vi "MLTraining.vi"(3 "model file (JSON)":path, 8 "Save model file as":string="model.json", 9 "model to train":T7(ring), 10 "Label setting":T2={"with label column?"=TRUE, "label column index"=-1}, 11 "training data file (CSV)":path) -> (0 "error out":errorcluster, 1 "feature trend":dbl[][](graph))   [LabVIEW 2017, in "MachineLearning.lvlib"]
doc: "Demonstrates how to find the optimal set of hyperparameters of the specific algorithm among SVM, Neural Network and Logistic Regression by grid search."
uses:
  MachineLearning.lvlib
  TypeDefs/Label Setting.ctl
  <vilib>/addons/AML/Classification/SVM/Controls/aml_SVM Grid Configuration.ctl
  <vilib>/addons/AML/Classification/SVM/Controls/aml_SVM Type.ctl
  <vilib>/addons/AML/Classification/SVM/Controls/aml_SVM Kernel Type.ctl
  <vilib>/addons/AML/Classification/Neural Network/Controls/aml_Neural Network Parameter Grid.ctl
  <vilib>/addons/AML/Classification/Neural Network/Controls/aml_Hidden Layer Type.ctl
  <vilib>/addons/AML/Classification/Neural Network/Controls/aml_Output Layer Type.ctl
  <vilib>/addons/AML/Classification/Neural Network/Controls/aml_NN Cost Function Type.ctl
  <vilib>/addons/AML/Classification/Logistic Regression/Controls/aml_Logistic Regression Parameters Grid.ctl
  <vilib>/addons/AML/Classification/SVM/Classes/AML SVM.lvclass/AML SVM.ctl
  <vilib>/addons/AML/Classification/Neural Network/Classes/AML Neural Network.lvclass/AML Neural Network.ctl
  <vilib>/addons/AML/Classification/Logistic Regression/Classes/AML Logistic Regression.lvclass/AML Logistic Regression.ctl
  <vilib>/addons/AML/Classification/SVM/Classes/aml_Read SVM Parameter.vi
  <vilib>/addons/AML/Classification/Neural Network/Classes/aml_Read Neural Network Parameter.vi
  <vilib>/addons/AML/Classification/Logistic Regression/Classes/aml_Read LR Parameters.vi
  <vilib>/addons/AML/Classification/SVM/Classes/AML SVM.lvclass
  C:/Program Files (x86)/National Instruments/LabVIEW 2017/vi.lib/addons/AML/Classification/Common/Classes/AML Classification.lvclass
  <vilib>/addons/AML/Classification/Neural Network/Classes/AML Neural Network.lvclass
  <vilib>/addons/AML/Classification/Logistic Regression/Classes/AML Logistic Regression.lvclass
  <vilib>/addons/AML/Classification/Initialize Classification Model (LR, Search).vi
  <vilib>/addons/AML/Classification/Initialize Classification Model (NN, Search).vi
  <vilib>/addons/AML/Classification/Initialize Classification Model (SVM, Search).vi
  <vilib>/addons/AML/Data/Load Training Data (2D Array).vi
  <vilib>/addons/AML/Analytics and Machine Learning.lvlib
panel:
  in  "Tab Control":T1(tab)
  in  "Tab Control 2":T3(tab)
  out "coef0":dbl
  out "gamma":dbl
  out "degree":i32
  out "nu":dbl
  out "c":dbl
  out "kernel type":enum32{"Linear", "Polynomial", "RBF", "Sigmoid"}(ring)
  out "SVM type":enum32{"C_SVC", "NU_SVC"}(ring)
  in  "hyperparameter optimization (SVM)":T4={"hyperparameter search method"=enum."Exhaustive search", "number of searchings"=1, "evaluation metric"=enum."Accuracy"} caption="hyperparameter optimization"
  in  "degree":i32[](array[numeric])=[3, 5]
  in  "nu":dbl[](array[numeric])=[0.3, 0.5]
  in  "c":dbl[](array[numeric])=[0.1, 1.0]
  in  "kernel type":T5(array[ring])=[enum."Linear", enum."Polynomial", enum."RBF", enum."Sigmoid"]
  in  "SVM type":enum32{"C_SVC", "NU_SVC"}[](array[ring])=[enum."C_SVC", enum."NU_SVC"]
  in  "gamma":dbl[](array[numeric])=[0.2, 0.5]
  in  "coef0":dbl[](array[numeric])=[0.0, 1.0]
  out "metrics (cross validation)":T6
  out "output layer type":enum16{"Sigmoid", "Softmax"}(ring)
  out "cost function type":enum16{"Quadratic", "Cross-entropy"}(ring)
  out "hidden layer type":enum16{"Sigmoid", "Tanh", "ReLU"}(ring)
  out "number of hidden neurons":i32
  in  "hyperparameter optimization (NN)":T4={"hyperparameter search method"=enum."Exhaustive search", "number of searchings"=1, "evaluation metric"=enum."Accuracy"} caption="hyperparameter optimization"
  in  "number of hidden neurons":i32[](array[numeric])=[5, 10]
  in  "hidden layer type":enum16{"Sigmoid", "Tanh", "ReLU"}[](array[ring])=[enum."Sigmoid", enum."Tanh", enum."ReLU"]
  in  "output layer type":enum16{"Sigmoid", "Softmax"}[](array[ring])=[enum."Sigmoid", enum."Softmax"]
  in  "cost function type":enum16{"Quadratic", "Cross-entropy"}[](array[ring])=[enum."Quadratic", enum."Cross-entropy"]
  out "metrics (cross validation)":T6
  out "max iteration":i32
  out "tolerance":dbl
  in  "tolerance":dbl[](array[numeric])=[0.001, 0.0001]
  in  "max iteration":i32[](array[numeric])=[500, 1000]
  in  "hyperparameter optimization (LR)":T4={"hyperparameter search method"=enum."Exhaustive search", "number of searchings"=1, "evaluation metric"=enum."Accuracy"} caption="hyperparameter optimization"
  out "metrics (cross validation)":T6
  # "Optimized Hyperparameters"
  # "Optimized Hyperparameters"
  # "Optimized Hyperparameters"
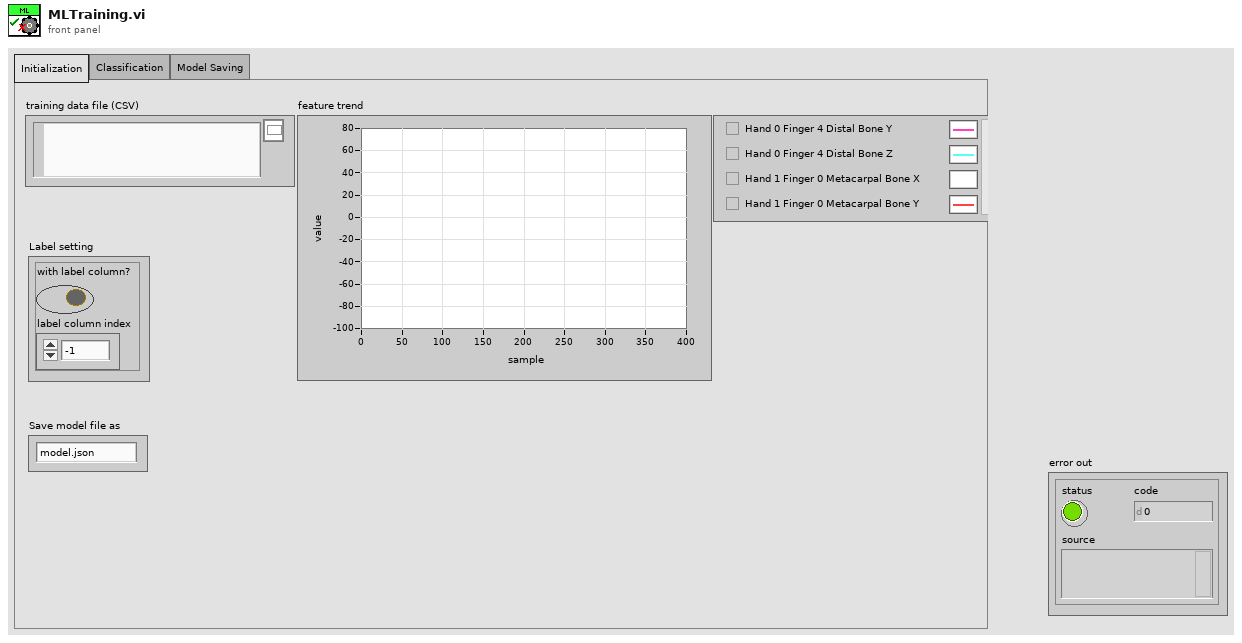
[diagram p1: front panel]
types:
  T1 = enum32{"Initialization", "Classification", "Model Saving"}
  T2 = typedef "MachineLearning.lvlib/Label Setting.ctl" = cluster{"with label column?":bool, "label column index":i32}
  T3 = enum32{"SVM", "Neural Network", "Logistic Regression"}
  T4 = cluster{"hyperparameter search method":enum16{"Exhaustive search", "Random search"}, "number of searchings":i32, "evaluation metric":enum16{"Accuracy", "Precision", "Recall", "F1 score"}}
  T5 = enum32{"Linear", "Polynomial", "RBF", "Sigmoid"}[]
  T6 = cluster{"accuracy":dbl, "precision":dbl, "recall":dbl, "f1 score":dbl}
  T7 = enum16{"SVM", "Neural Network", "Logistic Regression"}
  T8 = typedef "Analytics and Machine Learning.lvlib/aml_Logistic Regression Parameters Grid.ctl" = cluster{"tolerance":dbl[], "max iteration":i32[]}
  T9 = typedef "Analytics and Machine Learning.lvlib/aml_Neural Network Parameter Grid.ctl" = cluster{"number of hidden neurons":i32[], "hidden layer type":T10[], "output layer type":T11[], "cost function type":T12[], "tolerance":dbl[], "max iteration":i32[]}
  T10 = typedef "Analytics and Machine Learning.lvlib/aml_Hidden Layer Type.ctl" = enum16{"Sigmoid", "Tanh", "ReLU"}
  T11 = typedef "Analytics and Machine Learning.lvlib/aml_Output Layer Type.ctl" = enum16{"Sigmoid", "Softmax"}
  T12 = typedef "Analytics and Machine Learning.lvlib/aml_NN Cost Function Type.ctl" = enum16{"Quadratic", "Cross-entropy"}
  T13 = typedef "Analytics and Machine Learning.lvlib/aml_SVM Grid Configuration.ctl" = cluster{"SVM type":T14[], "c":dbl[], "nu":dbl[], "kernel settings":cluster{"type":T15[], "degree":i32[], "gamma":dbl[], "coef0":dbl[]}, "weighted c":cluster{"label":i32, "weight":dbl}[], "tolerance":dbl, "max iteration":i32}
  T14 = typedef "Analytics and Machine Learning.lvlib/aml_SVM Type.ctl" = enum32{"C_SVC", "NU_SVC"}
  T15 = typedef "Analytics and Machine Learning.lvlib/aml_SVM Kernel Type.ctl" = enum32{"Linear", "Polynomial", "RBF", "Sigmoid"}
  T16 = enum16{"open", "replace", "create", "open or create", "replace or create", "replace or create with confirmation"}
  T17 = typedef "Analytics and Machine Learning.lvlib/aml_Model Metrics.ctl" = cluster{"accuracy":dbl, "precision":dbl, "recall":dbl, "f1 score":dbl}
  T18 = typedef "Analytics and Machine Learning.lvlib/aml_SVM Parameters.ctl" = cluster{"SVM type":T14, "c":dbl, "nu":dbl, "kernel settings":T19, "weighted c":cluster{"label":i32, "weight":dbl}[], "tolerance":dbl, "max iteration":i32}
  T19 = typedef "Analytics and Machine Learning.lvlib/aml_SVM Kernel Settings.ctl" = cluster{"type":T15, "degree":i32, "gamma":dbl, "coef0":dbl}
  T20 = typedef "Analytics and Machine Learning.lvlib/aml_Neural Network Parameter.ctl" = cluster{"number of hidden neurons":i32, "hidden layer type":T10, "output layer type":T11, "cost function type":T12, "tolerance":dbl, "max iteration":i32}
  T21 = typedef "Analytics and Machine Learning.lvlib/aml_Logistic Regression Parameters.ctl" = cluster{"tolerance":dbl, "max iteration":i32}
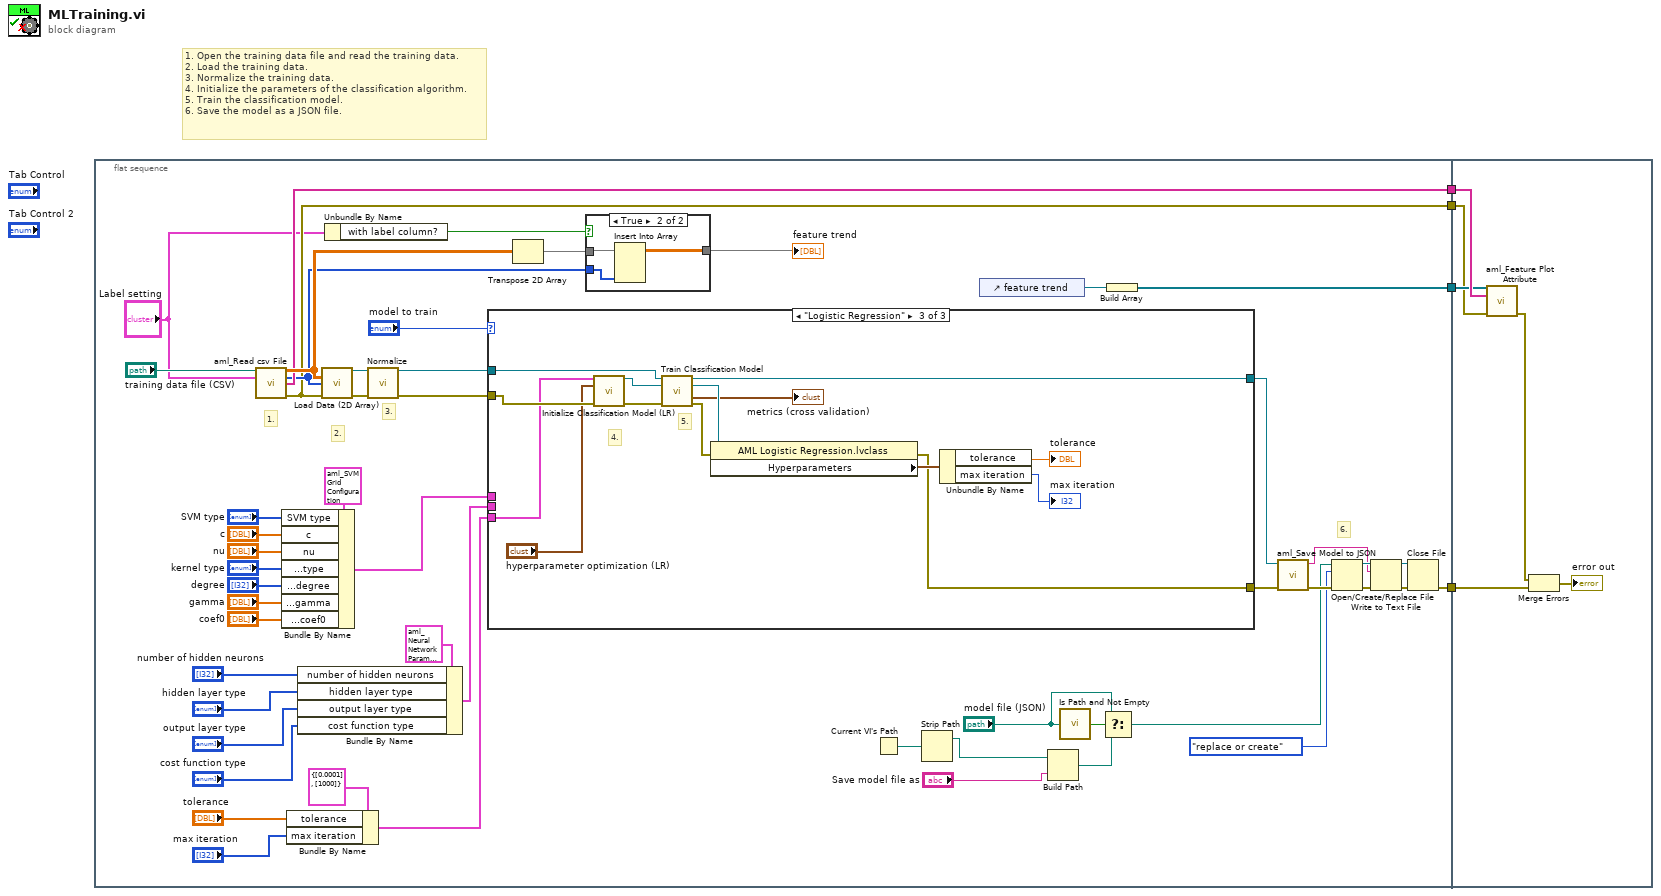
[diagram p0: block diagram]
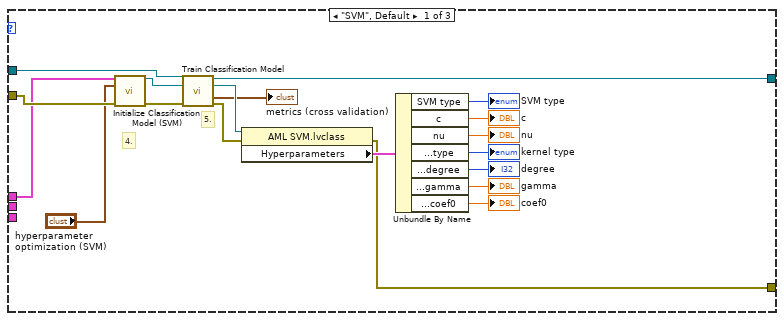
[diagram p3: hidden frame]
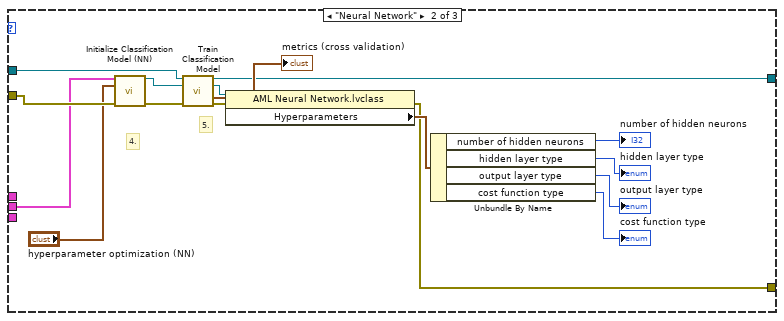
[diagram p4: hidden frame]
diagram:
  # "1. Open the training data file and read the training data.\n2. Load the training data.\n3. Normalize the training data.\n4. Initialize the parameters of the classification algorithm.\n5. Train the classification model.\n6. Save the model as a JSON file."
  n1 = flat-sequence {
    tunnel: [w48] -> w4
    tunnel: [w47] -> w3
    tunnel: [w39] -> w2
    tunnel: [w10] -> w1
    tunnel: w4 -> [w115]
    tunnel: w3 -> [w112]
    tunnel: w2 -> [w110]
    tunnel: w1 -> [w111]
    frame #0 {
      # "6."
      # "3."
      # "2."
      # "1."
      n2 = call <vilib>:"aml_Read csv File.vi"("csv file path"="training data file (CSV)", "Label setting"="Label setting") -> ("data"=w55:dbl[][], "data label"=w12:i32[], "feature names"=w48:string[], "error out"=w10:errorcluster)  [unwired: 10 in]
      n3 = Bundle By Name(cluster=T13 {"SVM type"=[enum."C_SVC"], "c"=[1.0], "nu"=[0.5], "kernel settings"={"type"=[enum."Linear"], "degree"=[3], "gamma"=[0.5], "coef0"=[0.0]}, "weighted c"=[], "tolerance"=0.001, "max iteration"=100000} ("hyperparameter grids"), "SVM type"="SVM type", "c"="c", "nu"="nu", "kernel settings.type"="kernel type", "kernel settings.degree"="degree", "kernel settings.gamma"="gamma", "kernel settings.coef0"="coef0") -> (w27:T13)
      n4 = Bundle By Name(cluster=T8 {"tolerance"=[0.0001], "max iteration"=[1000]} ("hyperparameter grids"), "tolerance"="tolerance", "max iteration"="max iteration") -> (w17:T8)
      n5 = Bundle By Name(cluster=T9 {"number of hidden neurons"=[5], "hidden layer type"=[enum."Sigmoid"], "output layer type"=[enum."Sigmoid"], "cost function type"=[enum."Quadratic"], "tolerance"=[0.0001], "max iteration"=[1000]} ("hyperparameter grids"), "number of hidden neurons"="number of hidden neurons", "hidden layer type"="hidden layer type", "output layer type"="output layer type", "cost function type"="cost function type") -> (w21:T9)
      n6 = call-poly <vilib>:"Load Data (2D Array).vi"("data"=w55, "data labels"=w12, "error in (no error)"=w10) -> ("model out"=w54:refnum<class "AML Analytics Model.lvclass">, "error out"=w53:errorcluster)  [unwired: 11 in]
      n7 = Unbundle By Name("Label setting") -> ("with label column?"=w11:bool)
      n8 = call <vilib>:"Normalize.vi"("model in"=w54, "error in (no error)"=w53) -> ("model out"=w36:refnum<class "AML Analytics Model.lvclass">, "error out"=w37:errorcluster)  [unwired: 11 in, 1 out]
      n9 = case shown="\"Logistic Regression\"" "model to train" {
        tunnel: w37 -> [w77 w94 w108]
        tunnel: w36 -> [w76 w95 w109]
        tunnel: w27 -> [w75 _ _]
        tunnel: w21 -> [_ w80 _]
        tunnel: w17 -> [_ _ w96]
        tunnel: [w63 w83 w99] -> w16
        tunnel: [w62 w82 w98] -> w15
        frame "SVM", Default {
          # "5."
          # "4."
          n10 = call-poly <vilib>:"Initialize Classification Model (SVM).vi"("hyperparameter grids"=w75, "hyperparameter optimization"="hyperparameter optimization (SVM)", "error in (no error)"=w77) -> ("untrained SVM model"=w78:refnum<class "AML SVM.lvclass">, "error out"=w79:errorcluster)  [unwired: 11 in]
          n11 = call <vilib>:"Train Classification Model.vi"("model in"=w76, "classification model info in"=w78, "error in (no error)"=w79) -> ("model out"=w63:refnum<class "AML Analytics Model.lvclass">, "classification model info out"=w74:refnum<class "AML SVM.lvclass">, "metrics"=→"metrics (cross validation)":T17, "error out"=w73:errorcluster)  [unwired: 8 in, 1 out]
          n12 = property class="AML SVM.lvclass"(reference=w74, error in=w73) -> (error out=w62:errorcluster, "Hyperparameters"=w72:T18)  [unwired: 1 out]
          n13 = Unbundle By Name(w72) -> ("SVM type"=→"SVM type":T14, "c"=→"c":dbl, "nu"=→"nu":dbl, "kernel settings.type"=→"kernel type":T15, "kernel settings.degree"=→"degree":i32, "kernel settings.gamma"=→"gamma":dbl, "kernel settings.coef0"=→"coef0":dbl)
        }
        frame "Neural Network" {
          # "5."
          # "4."
          n14 = call-poly <vilib>:"Initialize Classification Model (NN).vi"("hyperparameter grids"=w80, "hyperparameter optimization"="hyperparameter optimization (NN)", "error in (no error)"=w94) -> ("untrained neural network model"=w91:refnum<class "AML Neural Network.lvclass">, "error out"=w93:errorcluster)  [unwired: 11 in]
          n15 = call <vilib>:"Train Classification Model.vi"("model in"=w95, "classification model info in"=w91, "error in (no error)"=w93) -> ("model out"=w83:refnum<class "AML Analytics Model.lvclass">, "classification model info out"=w90:refnum<class "AML Neural Network.lvclass">, "metrics"=→"metrics (cross validation)":T17, "error out"=w89:errorcluster)  [unwired: 8 in, 1 out]
          n16 = property class="AML Neural Network.lvclass"(reference=w90, error in=w89) -> (error out=w82:errorcluster, "Hyperparameters"=w88:T20)  [unwired: 1 out]
          n17 = Unbundle By Name(w88) -> ("number of hidden neurons"=→"number of hidden neurons":i32, "hidden layer type"=→"hidden layer type":T10, "output layer type"=→"output layer type":T11, "cost function type"=→"cost function type":T12)
        }
        frame "Logistic Regression" {
          # "5."
          # "4."
          n18 = call-poly <vilib>:"Initialize Classification Model (LR).vi"("hyperparameter grids"=w96, "hyperparameter optimization"="hyperparameter optimization (LR)", "error in (no error)"=w108) -> ("untrained logistic regression model"=w106:refnum<class "AML Logistic Regression.lvclass">, "error out"=w107:errorcluster)  [unwired: 11 in]
          n19 = call <vilib>:"Train Classification Model.vi"("model in"=w109, "classification model info in"=w106, "error in (no error)"=w107) -> ("model out"=w99:refnum<class "AML Analytics Model.lvclass">, "classification model info out"=w105:refnum<class "AML Logistic Regression.lvclass">, "metrics"=→"metrics (cross validation)":T17, "error out"=w104:errorcluster)  [unwired: 8 in, 1 out]
          n20 = property class="AML Logistic Regression.lvclass"(reference=w105, error in=w104) -> (error out=w98:errorcluster, "Hyperparameters"=w103:T21)  [unwired: 1 out]
          n21 = Unbundle By Name(w103) -> ("tolerance"=→"tolerance":dbl, "max iteration"=→"max iteration":i32)
        }
      }
      n22 = Transpose 2D Array(2D array=w55) -> (transposed array=w13:dbl[][])
      n23 = case shown="True" w11 {
        tunnel: w12 -> [_ w59]
        tunnel: w13 -> [w57 w60]
        tunnel: [w57 w58] -> w9
        frame False {
        }
        frame True {
          n24 = Insert Into Array(array=w60, new element=w59) -> (w58:dbl[][])  [unwired: 2 in]
        }
      }
      "feature trend" <- w9
      n25 = Current VI's Path() -> (path=w49:path)
      n26 = Strip Path(path=w49) -> (stripped path=w6:path)  [unwired: 1 out]
      n27 = control-ref of="feature trend"() -> (w8:refnum<vi>)
      n28 = Build Path(base path=w6, name or relative path="Save model file as") -> (appended path=w50:path)
      n29 = call <vilib>:"Is Path and Not Empty.vi"("path"="model file (JSON)") -> ("Is Path and Not Empty?"=w52:bool)  [unwired: 4 in]
      n30 = Select(t="model file (JSON)", s=w52, f=w50) -> (s? t:f=w42:path)
      n31 = Build Array(w8) -> (w47:refnum<vi>[])
      n32 = call <vilib>:"aml_Save Model to JSON.vi"("error in (no error)"=w15, "model in"=w16) -> ("error out"=w44:errorcluster, "JSON string"=w38:string)  [unwired: 8 in]
      n33 = Open/Create/Replace File(file path (use dialog)=w42, error in=w44, operation (0:open)=T16."replace or create") -> (refnum out=w41:refnum<file>, error out=w45:errorcluster)  [unwired: 3 in, 1 out]
      n34 = Write to Text File(file (use dialog)=w41, text=w38, error in=w45) -> (refnum out=w40:refnum<file>, error out=w46:errorcluster)  [unwired: 1 in, 1 out]
      n35 = Close File(refnum=w40, error in=w46) -> (error out=w39:errorcluster)  [unwired: 1 out]
    }
    frame #1 {
      n36 = call <vilib>:"aml_Feature Plot Attribute.vi"("error in (no error)"=w111, "feature names"=w115, "appended array"=w112) -> ("error in (no error)"=w114:errorcluster)  [unwired: 8 in]
      n37 = Merge Errors(w114, w110) -> (→"error out":errorcluster)
    }
  }
